vi "Set position DSP402.vi"(8 "error in (no error)":errorcluster, 10 "Position units":i32, 11 "DSP402 in":refnum<class "DSP402.lvclass">) -> (0 "error out":errorcluster, 3 "DSP402 out":refnum<class "DSP402.lvclass">)   [LabVIEW 2024, in "canopen.lvlib" / "DSP402.lvclass"]
uses:
  DSP402.lvclass
  DSP402.lvclass/DSP402.ctl
  CANopen/Multiplexor.ctl
  CANopen Master.lvlib
  <userlib>/_OpenG.lib/error/error.llb/openg_error.lvlib
  Download DSP402 (U32).vi
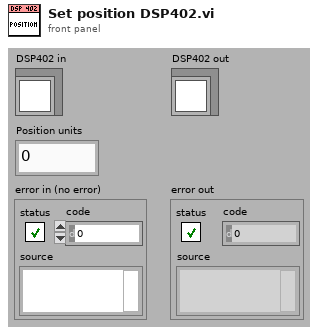
[diagram p1: front panel]
types:
  T1 = typedef "canopen.lvlib/DSP402.lvclass/DriveMode.ctl" = i8
  T2 = typedef "CANopen Master.lvlib/Multiplexor.ctl" = cluster{"Index":u16, "Sub-Index":u8}
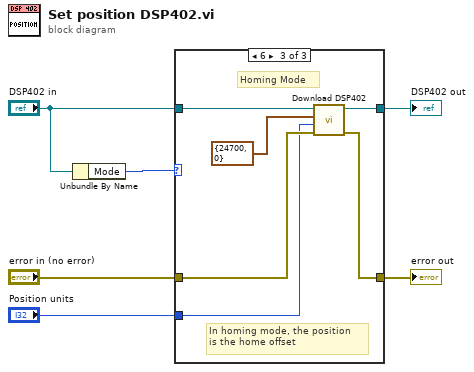
[diagram p0: block diagram]
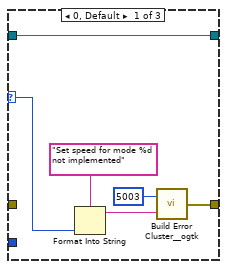
[diagram p2: hidden frame]
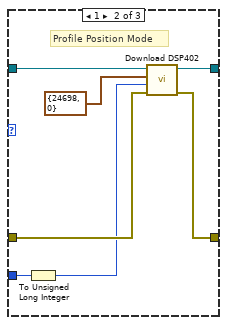
[diagram p3: hidden frame]
diagram:
  n1 = Unbundle By Name("DSP402 in") -> ("Mode"=w3:T1)
  n2 = case shown="6" w3 {
    selector: w3 -> [w9 _ _]
    tunnel: [w10 w19 w24] -> w4
    tunnel: "error in (no error)" -> [_ w18 w23]
    tunnel: "Position units" -> [_ w17 w22]
    tunnel: [w7 w13 w20] -> w2
    tunnel: "DSP402 in" -> [w7 w14 w21]
    frame 0, Default {
      n3 = Format Into String(format string="Set speed for mode %d not implemented", w9) -> (resulting string=w11:string)  [unwired: 2 in, 1 out]
      n4 = call <userlib>:"Build Error Cluster__ogtk.vi"("String to Prepend to source (\"\")"=w11, "code"=5003) -> ("error out"=w10:errorcluster)
    }
    frame 1 {
      # "Profile Position Mode"
      n5 = To Unsigned Long Integer(number=w17) -> (unsigned 32bit integer=w16:u32)
      n6 = call-poly "Download DSP402.vi"("error in (no error)"=w18, "Value"=w16, "Multiplexor"=T2 {"Index"=24698, "Sub-Index"=0}, "DSP402 in"=w14) -> ("error out"=w19:errorcluster, "DSP402 out"=w13:refnum<class "DSP402.lvclass">)  [unwired: 1 in, 1 out]
    }
    frame 6 {
      # "In homing mode, the position\nis the home offset"
      # "Homing Mode"
      n7 = call-poly "Download DSP402.vi"("error in (no error)"=w23, "Value"=w22, "Multiplexor"=T2 {"Index"=24700, "Sub-Index"=0}, "DSP402 in"=w21) -> ("error out"=w24:errorcluster, "DSP402 out"=w20:refnum<class "DSP402.lvclass">)  [unwired: 1 in, 1 out]
    }
  }
  "error out" <- w4
  "DSP402 out" <- w2
